vi "FTW-TransferClient-S3-ObjectURL.vi"(0 "Object Bucket":string, 1 "Object Key":string) -> (3 "Object URL":string)   [LabVIEW 2014, in "FTW-TransferClient-S3.lvclass"]
uses:
  FTW-TransferClient-S3.lvclass
panel:
  # "Inputs"
  # "Outputs"
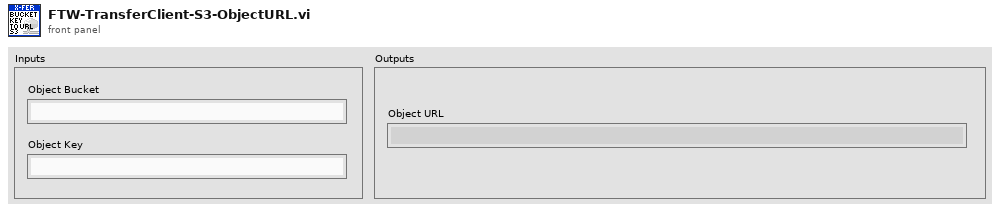
[diagram p1: front panel]
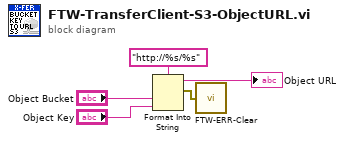
[diagram p0: block diagram]
diagram:
  n1 = Format Into String(format string="http://%s/%s", "Object Bucket", "Object Key") -> (resulting string=→"Object URL":string, error out=w1:errorcluster)  [unwired: 2 in]
  n2 = call "FTW-ERR-Clear.vi"("error to snuff"=w1) -> ()  [unwired: 1 out]
